vi "OCR_Setting_UI.vi"(6 "Analysis_Setting":T1={"PreProcess"=enum."*Algorithm*", "Parameter"=""}, 8 "error in (no error)":errorcluster, 9 "ProjectName":string="CDF", 10 "LstBox Refnum":refnum<vi>, 11 "Vision_Image":T4(plugin-control)) -> (0 "error out":errorcluster, 1 "Cancel?":bool, 3 "output cluster":T1={"PreProcess"=enum."*Algorithm*", "Parameter"=""})   [LabVIEW 2019]
uses:
  Controls/_UI Command Cluster/OCR_UI Command.ctl
  Controls/_UI Command Cluster/OCR_UI Command Array.ctl
  Controls/Analysis_Type.ctl
  Controls/OCR/Analysis_OCR_Setting Parameter.ctl
  Controls/Analysis_Setting.ctl
  Controls/V_Analysis_Type.ctl
  Ctrl/VisionProcessName.ctl
panel:
  in  "OCR_Setting":T3
  in  "OCRRun":bool
  in  "Done":bool
  in  "Cancel":bool
  in  "OCRTab":enum32{"Standard Setting", "Result"}(tab)
  in  "OCRLangAdd":bool
  in  "OCRLangRemove":bool
  in  "OCRSelectedLanaguage":i32(listbox)
  in  "OCRLanguage":u16(ring)
  out "OCR Result":string
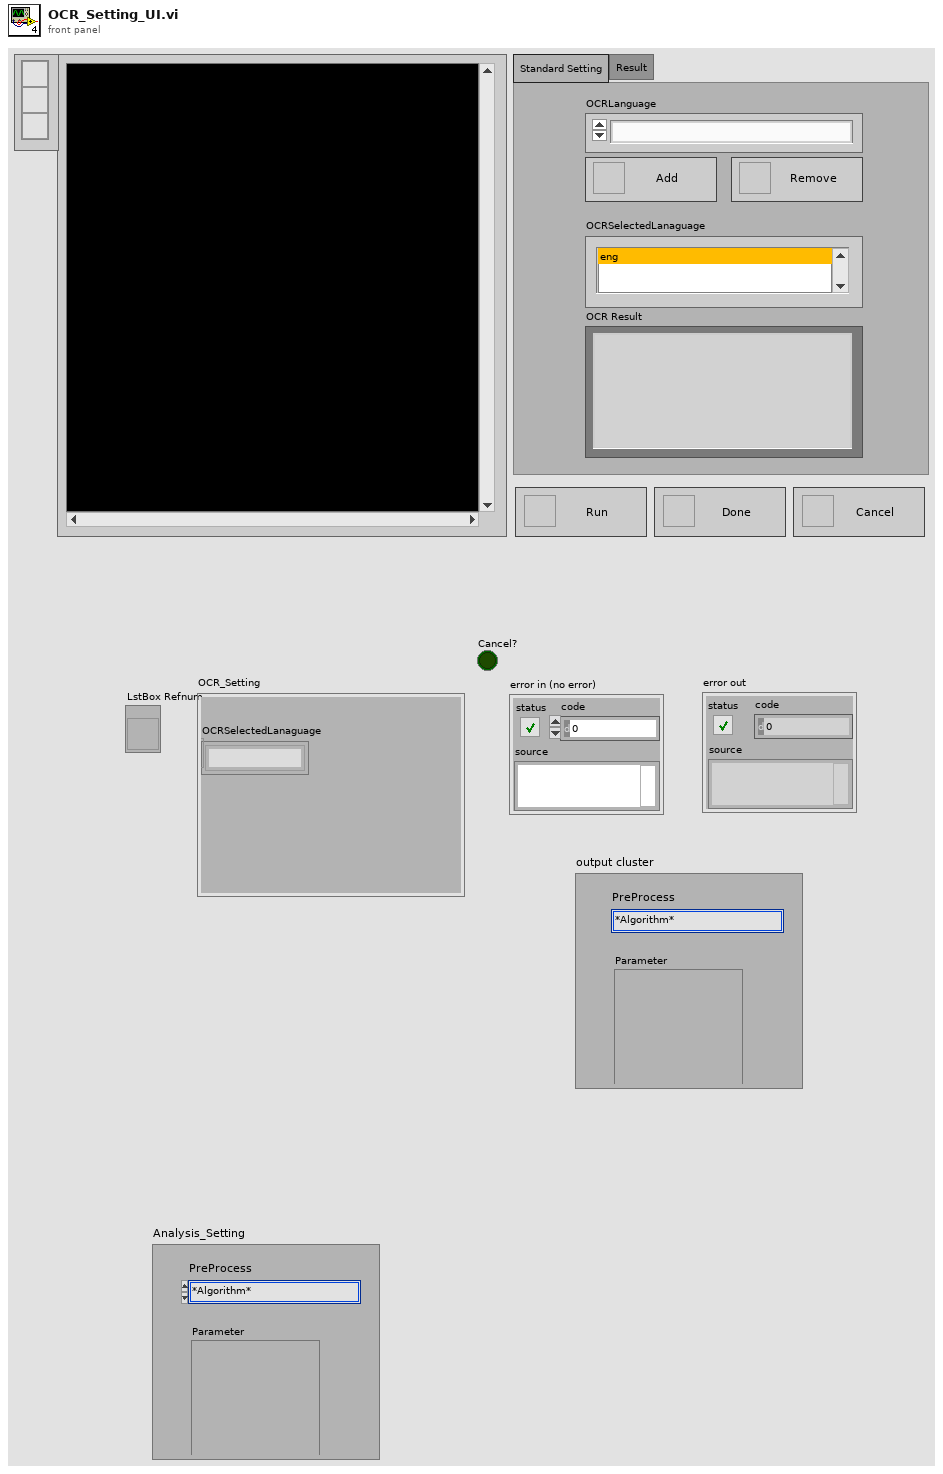
[diagram p1: front panel]
types:
  T1 = typedef "Analysis_Setting.ctl" = cluster{"PreProcess":T2, "Parameter":string}
  T2 = typedef "VisionProcessName.ctl" = enum16{"*CamParameter*", "CamAttributes", "*Preprocess*", "CG_Brightness", "C_Plane Extraction", "C_Threshold", "G_Lookup Table", "G_Threshold", "B_Image Inversion", "*Algorithm*", "CG_Histogram", "C_Color Matching", "C_Color Pattern Matching", "G_PatternMatch", "CG_Find Straight Edge", "CG_Adv. Find Straight Edge", "CG_Find Circular Edge", "G_Max Clamp", "G_Clamp (Rake)", "G_Pattern Matching"}
  T3 = typedef "Analysis_OCR_Setting Parameter.ctl" = cluster{"OCRSelectedLanaguage":string[]}
  T4 = typedef "IMAQ Image.ctl" = refnum<image>
  T5 = typedef "OCR_UI Command Array.ctl" = T6[]
  T6 = typedef "OCR_UI Command.ctl" = enum16{"Initialize", "Read Language Package", "Run", "Get Project ROI Name", "Done", "Cancel", "Add To Language", "Remove To Language", "Read Result", "Delete File", "Draw Overlay"}
  T7 = cluster{"Desired Font (Application)":enum16{"User-specified Font", "Application Font", "System Font", "Dialog Font"}, "[User-specified Font]":cluster{"Font Name":string, "Size":i16, "Strikeout?":bool, "Italic?":bool, "Underline?":bool, "Outline?":bool, "Shadow?":bool, "Bold?":bool, "Rotation Angle":dbl}, "Horizontal Alignment":i16, "Vertical Alignment":i16}
  T8 = typedef "Analysis_Type.ctl" = u16
  T9 = typedef "Analysis_Setting.ctl" = cluster{"PreProcess":T10, "Parameter":string}
  T10 = typedef "V_Analysis_Type.ctl" = enum16{"None", "C_Color Pattern Matching", "G_PatternMatching", "G_ShapeDectect", "G_GeometricMatch", "B_Area Check"}
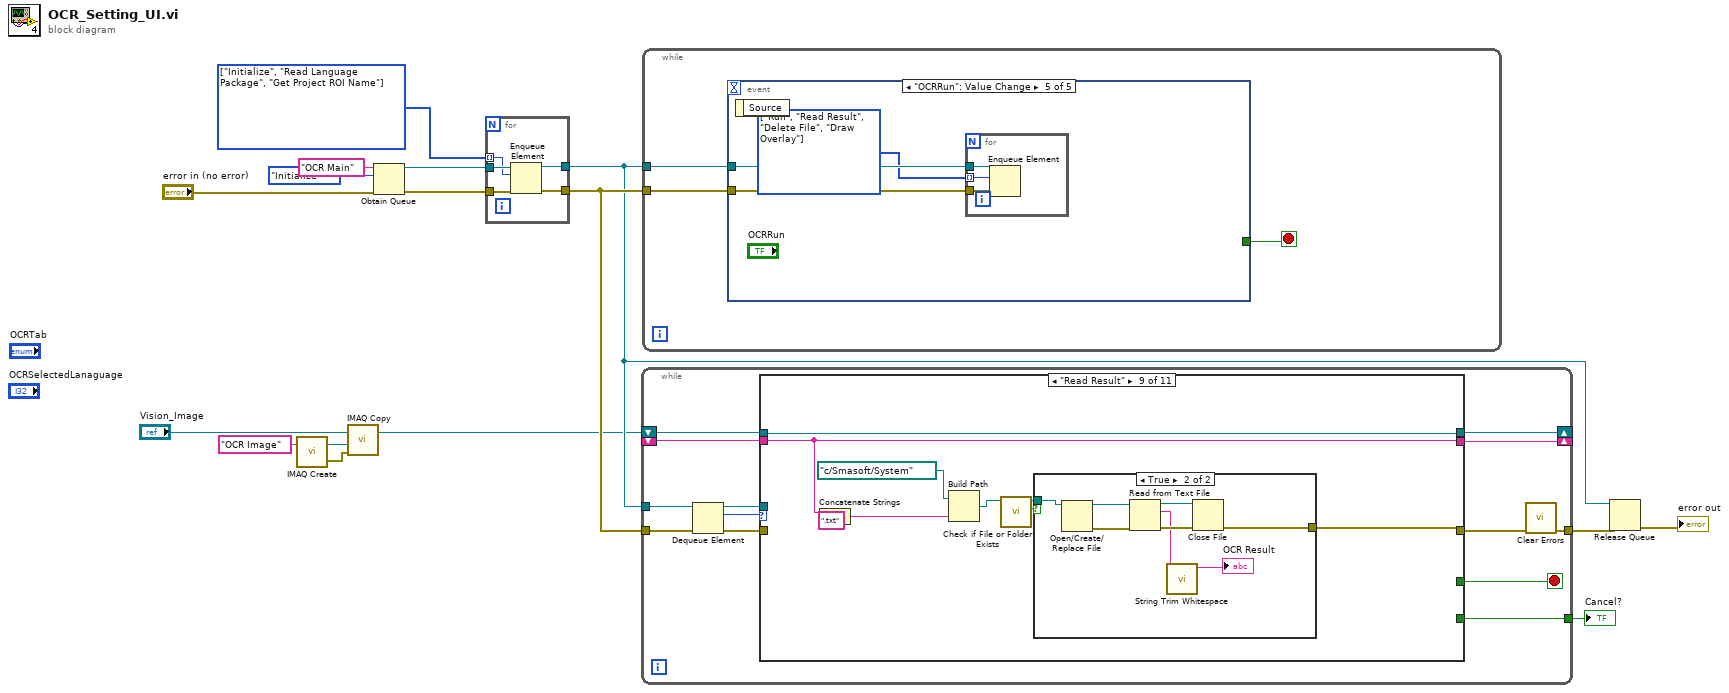
[diagram p0: block diagram]
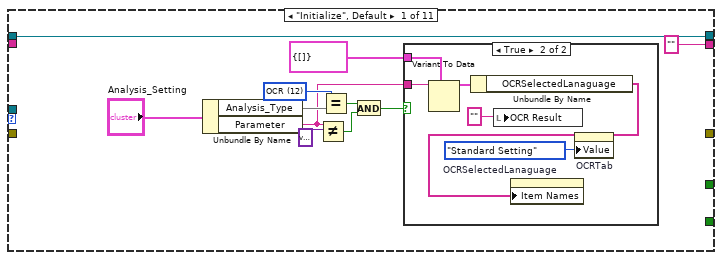
[diagram p2: hidden frame]
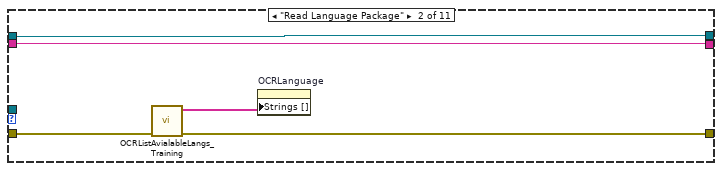
[diagram p4: hidden frame]
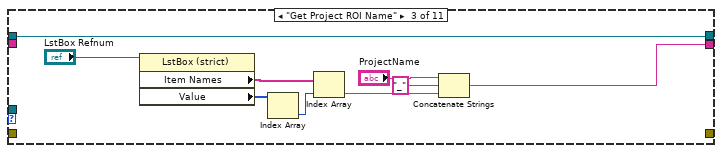
[diagram p5: hidden frame]
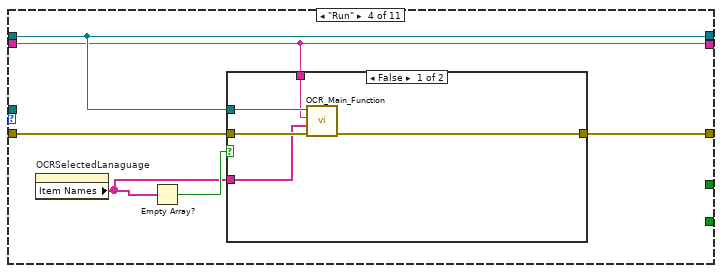
[diagram p6: hidden frame]
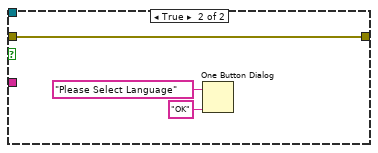
[diagram p7: hidden frame]
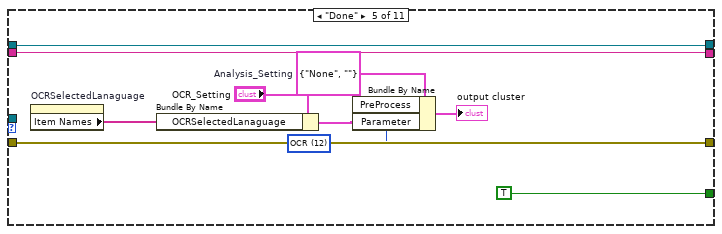
[diagram p8: hidden frame]
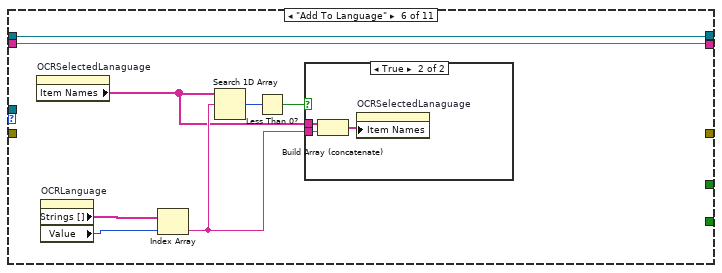
[diagram p9: hidden frame]
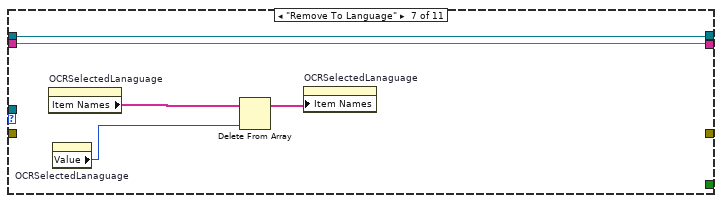
[diagram p11: hidden frame]
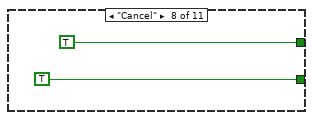
[diagram p12: hidden frame]
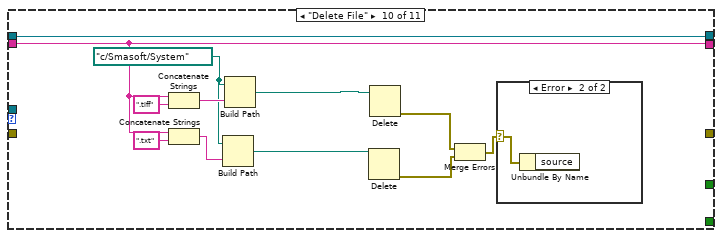
[diagram p14: hidden frame]
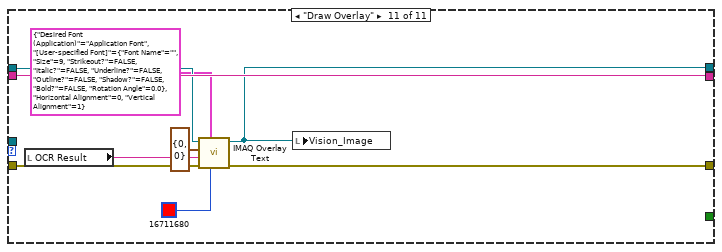
[diagram p16: hidden frame]
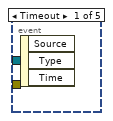
[diagram p17: hidden frame]
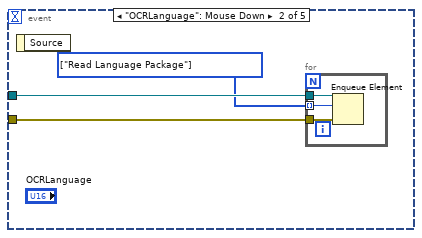
[diagram p18: hidden frame]
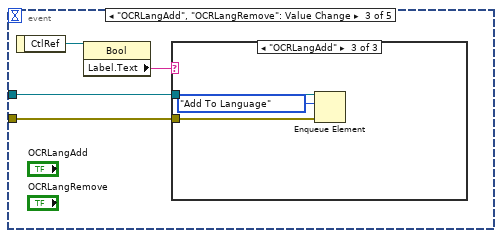
[diagram p19: hidden frame]
diagram:
  w10 = T5 [enum."Initialize", enum."Read Language Package", enum."Get Project ROI Name"] items=["Initialize", "Read Language Package", "Run", "Get Project ROI Name", "Done", "Cancel", "Add To Language", "Remove To Language", "Read Result", "Delete File", "Draw Overlay"] ("element")
  n1 = call "IMAQ Create"("Image Name"="OCR Image") -> ("New Image"=w5:T4, "error out"=w4:errorcluster)  [unwired: 4 in]
  n2 = call "IMAQ Copy"("error in (no error)"=w4, "Image Dst"=w5, "Image Src"="Vision_Image") -> ("Image Dst Out"=w2:T4)  [unwired: 3 in, 1 out]
  n3 = Obtain Queue(name (unnamed)="OCR Main", element data type=OCR_UI_Command."Initialize" ("OCR_UI Command"), error in (no error)="error in (no error)") -> (queue out=w12:refnum<queue>, error out=w11:errorcluster)  [unwired: 2 in, 1 out]
  n4 = for {
    tunnel: [w21] -> w16
    tunnel: [w20] -> w9
    tunnel: w12 -> [w19]
    tunnel: w11 -> [w18]
    tunnel: w10 -> [w17] mode=indexing
    n5 = Enqueue Element(queue=w19, element=w17, error in (no error)=w18) -> (queue out=w20:refnum<queue>, error out=w21:errorcluster)  [unwired: 1 in, 1 out]
  }
  n6 = while {
    tunnel: w16 -> [w34]
    tunnel: w9 -> [w33]
    tunnel: [w23] -> w1
    shift-right: [w27] -> _
    shift-left: _ -> [w26]
    shift-right: [w25] -> _
    shift-left: w2 -> [w28]
    tunnel: [w24] -> w7
    stop <- w29 stop-if-true
    n7 = Dequeue Element(queue=w33, error in (no error)=w34) -> (queue out=w32:refnum<queue>, element=w30:T6, error out=w31:errorcluster)  [unwired: 1 in, 1 out]
    n8 = case shown="\"Read Result\"" w30 {
      tunnel: w32 -> [_ _ _ _ _ _ _ _ _ _ _]
      tunnel: w31 -> [_ w53 _ w71 w82 _ _ _ _ _ w144]
      tunnel: [_ w52 _ w70 w82 _ _ _ w108 _ w143] -> w22
      tunnel: [_ _ _ _ TRUE _ _ TRUE _ _ _] -> w29
      tunnel: w28 -> [w45 w56 w57 w69 w89 w95 w102 _ w116 w136 w139]
      tunnel: ["" w55 w58 w68 w88 w94 w101 _ w114 w133 w146] -> w27
      tunnel: w26 -> [_ w55 _ w68 w88 w94 w101 _ w114 w133 w146]
      tunnel: [w45 w56 w57 w69 w89 w95 w102 _ w116 w136 w140] -> w25
      tunnel: [_ _ _ _ _ _ _ TRUE _ _ _] -> w24
      frame "Initialize", Default {
        w40 = T8 12 items=["None", "PatternMatch", "Edge Detection", "Barcode 1D", "Barcode 2D", "Clamp", "Clamp MAX", "Particle", "Histogram", "Straight Edge", "Circle", "Shape Detect", "OCR", "Contour", "ColorMatch"] ("x")
        n9 = Unbundle By Name("Analysis_Setting") -> ("Analysis_Type"=w41, "Parameter"=w35:string)
        n10 = Not Equal?(x=w35, y=variant) -> (x != y?=w38:bool)
        n11 = Equal?(x=w40, y=w41) -> (x = y?=w39:bool)
        n12 = And(x=w39, y=w38) -> (x .and. y?=w37:bool)
        n13 = case shown="True" w37 {
          tunnel: T3 {"OCRSelectedLanaguage"=[]} ("OCR_Setting Parameter") -> [_ w50]
          tunnel: w35 -> [_ w49]
          frame False {
          }
          frame True {
            n14 = Variant To Data(type=w50, Variant=w49) -> (data=w51:T3)  [unwired: 1 in, 1 out]
            n15 = Unbundle By Name(w51) -> ("OCRSelectedLanaguage"=w48:string[])
            n16 = local write "OCR Result"("") -> ()
            n17 = property on="OCRSelectedLanaguage" class="LstBox (strict)"("Item Names"=w48) -> ()  [unwired: 2 in, 2 out]
            n18 = property on="OCRTab" class="TabCtl (strict)"("Value"=enum32{"Standard Setting", "Result"}."Standard Setting" ("OCRTab")) -> ()  [unwired: 2 in, 2 out]
          }
        }
      }
      frame "Read Language Package" {
        n19 = call "OCRListAvialableLangs_Training.vi"("error in (no error)"=w53) -> ("error out"=w52:errorcluster, "Langs"=w54:string[])  [unwired: 9 in]
        n20 = property on="OCRLanguage" class="Ring (strict)"("Strings []"=w54) -> ()  [unwired: 2 in, 2 out]
      }
      frame "Get Project ROI Name" {
        n21 = property class="LstBox (strict)"(reference="LstBox Refnum") -> ("Item Names"=w60:string[], "Value"=w59:i32[])  [unwired: 1 in, 2 out]
        n22 = Index Array(array=w59) -> (element=w62:i32)  [unwired: 1 in]
        n23 = Index Array(array=w60, index=w62) -> (element=w63:string)
        n24 = Concatenate Strings("ProjectName", "_" ("string"), w63) -> (w58:string)
      }
      frame "Run" {
        n25 = property on="OCRSelectedLanaguage" class="LstBox (strict)"() -> ("Item Names"=w66:string[])  [unwired: 2 in, 2 out]
        n26 = Empty Array?(array=w66) -> (empty?=w67:bool)
        n27 = case shown="False" w67 {
          tunnel: w71 -> [w76 w77]
          tunnel: [w75 w77] -> w70
          tunnel: w69 -> [w74 _]
          tunnel: w68 -> [w73 _]
          tunnel: w66 -> [w72 _]
          frame False {
            n28 = call "OCR_Main_Function.vi"("error in (no error)"=w76, "Item Names"=w72, "String"=w73, "Refnum in"=w74) -> ("error out"=w75:errorcluster)  [unwired: 7 in]
          }
          frame True {
            n29 = One Button Dialog(message="Please Select Language", button name ("OK")="OK") -> ()  [unwired: 1 out]
          }
        }
      }
      frame "Done" {
        w80 = T9 {"PreProcess"=enum."None", "Parameter"=""}  # Analysis_Setting
        w81 = T8 12 items=["None", "PatternMatch", "Edge Detection", "Barcode 1D", "Barcode 2D", "Clamp", "Clamp MAX", "Particle", "Histogram", "Straight Edge", "Circle", "Shape Detect", "OCR", "Contour", "ColorMatch"] ("Analysis_Type")
        n30 = property on="OCRSelectedLanaguage" class="LstBox (strict)"() -> ("Item Names"=w85:string[])  [unwired: 2 in, 2 out]
        n31 = Bundle By Name(cluster="OCR_Setting", "OCRSelectedLanaguage"=w85) -> (w86:T3)
        n32 = Bundle By Name(cluster=w80, "PreProcess"=w81, "Parameter"=w86) -> (→"output cluster":T9)
      }
      frame "Add To Language" {
        n33 = property on="OCRSelectedLanaguage" class="LstBox (strict)"() -> ("Item Names"=w90:string[])  [unwired: 2 in, 2 out]
        n34 = property on="OCRLanguage" class="Ring (strict)"() -> ("Strings []"=w96:string[], "Value"=w97:u16)  [unwired: 2 in, 2 out]
        n35 = Index Array(array=w96, index=w97) -> (element=w93:string)
        n36 = Search 1D Array(1D array=w90, element=w93) -> (index of element=w92:i32)  [unwired: 1 in]
        n37 = Less Than 0?(x=w92) -> (x < 0?=w91:bool)
        n38 = case shown="True" w91 {
          tunnel: w93 -> [_ w99]
          tunnel: w90 -> [_ w98]
          frame False {
          }
          frame True {
            n39 = Build Array (concatenate)(w98, w99) -> (w100:string[])
            n40 = property on="OCRSelectedLanaguage" class="LstBox (strict)"("Item Names"=w100) -> ()  [unwired: 2 in, 2 out]
          }
        }
      }
      frame "Remove To Language" {
        n41 = property on="OCRSelectedLanaguage" class="LstBox (strict)"() -> ("Item Names"=w105:string[])  [unwired: 2 in, 2 out]
        n42 = property on="OCRSelectedLanaguage" class="LstBox (strict)"() -> ("Value"=w104:i32)  [unwired: 2 in, 2 out]
        n43 = Delete From Array(array=w105, index=w104) -> (array with subset deleted=w103:string[])  [unwired: 1 in, 1 out]
        n44 = property on="OCRSelectedLanaguage" class="LstBox (strict)"("Item Names"=w103) -> ()  [unwired: 2 in, 2 out]
      }
      frame "Cancel" {
      }
      frame "Read Result" {
        n45 = Concatenate Strings(w114, ".txt" ("string")) -> (w112:string)
        n46 = Build Path(base path=path "c:/Smasoft/System", name or relative path=w112) -> (appended path=w111:path)
        n47 = call <vilib>:"Check if File or Folder Exists.vi"("path"=w111) -> ("file or folder exists?"=w110:bool, "dup path"=w109:path)  [unwired: 8 in, 1 out]
        n48 = case shown="True" w110 {
          tunnel: w109 -> [_ w120]
          tunnel: [_ w119] -> w108
          frame False {
          }
          frame True {
            n49 = Open/Create/Replace File(file path (use dialog)=w120) -> (refnum out=w124:refnum<file>, error out=w123:errorcluster)  [unwired: 5 in, 1 out]
            n50 = Read from Text File(file (use dialog)=w124, error in=w123) -> (refnum out=w122:refnum<file>, text=w118:string, error out=w121:errorcluster)  [unwired: 2 in, 1 out]
            n51 = call "String Trim Whitespace.vi"("String"=w118) -> ("*(type *) &x"=→"OCR Result":string)  [unwired: 10 in]
            n52 = Close File(refnum=w122, error in=w121) -> (error out=w119:errorcluster)  [unwired: 1 out]
          }
        }
      }
      frame "Delete File" {
        w131 = path "c:/Smasoft/System"
        n53 = Concatenate Strings(w133, ".tiff" ("string")) -> (w134:string)
        n54 = Concatenate Strings(w133, ".txt" ("string")) -> (w130:string)
        n55 = Build Path(base path=w131, name or relative path=w130) -> (appended path=w125:path)
        n56 = Build Path(base path=w131, name or relative path=w134) -> (appended path=w126:path)
        n57 = Delete(path (use dialog)=w125) -> (error out=w128:errorcluster)  [unwired: 4 in, 2 out]
        n58 = Delete(path (use dialog)=w126) -> (error out=w129:errorcluster)  [unwired: 4 in, 2 out]
        n59 = Merge Errors(w129, w128) -> (w127:errorcluster)
        n60 = case shown="Error" w127 {
          selector: w127 -> [_ w137]
          frame No Error {
          }
          frame Error {
            n61 = Unbundle By Name(w137) -> ()  [unwired: 1 out]
          }
        }
      }
      frame "Draw Overlay" {
        n62 = local read "OCR Result"() -> (w145:string)
        n63 = call "IMAQ Overlay Text"("Text Color (black)"=u32 16711680, "Font, Size & Style"=T7 {"Desired Font (Application)"=enum."Application Font", "[User-specified Font]"={"Font Name"="", "Size"=9, "Strikeout?"=FALSE, "Italic?"=FALSE, "Underline?"=FALSE, "Outline?"=FALSE, "Shadow?"=FALSE, "Bold?"=FALSE, "Rotation Angle"=0.0}, "Horizontal Alignment"=0, "Vertical Alignment"=1}, "error in (no error)"=w144, "String"=w145, "Origin"=cluster{"X":i32, "Y":i32} {"X"=0, "Y"=0}, "Image"=w139) -> ("error out"=w143:errorcluster, "Image Out"=w140:T4)  [unwired: 4 in]
        n64 = local write "Vision_Image"(w140) -> ()
      }
    }
    n65 = call <vilib>:"Clear Errors.vi"("error in (no error)"=w22) -> ("error out"=w23:errorcluster)  [unwired: 5 in, 1 out]
  }
  "Cancel?" <- w7
  n66 = while {
    tunnel: w16 -> [w148]
    tunnel: w9 -> [w149]
    stop <- w147 stop-if-true
    n67 = event shown="[4] \"OCRRun\": Value Change" {
      selector: _ -> [_ _ _ _ _]
      dyn-events: _ -> [_ _ _ _ _]
      timeout: _ -> [_ _ _ _ _]
      tunnel: w149 -> [_ w152 w157 w168 w181]
      tunnel: w148 -> [_ w151 w156 w167 w180]
      tunnel: [_ _ _ w166 _] -> w147
      event Timeout {
        n68 = event-data() -> ()  [unwired: 1 in, 3 out]
      }
      event "OCRLanguage": Mouse Down {
        w150 = T5 [enum."Read Language Package"] items=["Initialize", "Read Language Package", "Run", "Get Project ROI Name", "Done", "Cancel", "Add To Language", "Remove To Language", "Read Result", "Delete File", "Draw Overlay"] ("OCR_UI Command Array")
        n69 = event-data() -> ()  [unwired: 1 in, 1 out]
        n70 = for {
          tunnel: w152 -> [w155]
          tunnel: w151 -> [w154]
          tunnel: w150 -> [w153] mode=indexing
          n71 = Enqueue Element(queue=w155, element=w153, error in (no error)=w154) -> ()  [unwired: 1 in, 3 out]
        }
      }
      event "OCRLangAdd", "OCRLangRemove": Value Change {
        n72 = event-data() -> ("CtlRef"=w159:refnum<vi>)  [unwired: 1 in]
        n73 = property class="Bool"(reference=w159) -> ("Label.Text"=w158:string)  [unwired: 1 in, 2 out]
        n74 = case shown="\"OCRLangAdd\"" w158 {
          tunnel: w157 -> [_ w162 w165]
          tunnel: w156 -> [_ w161 w164]
          frame Default {
          }
          frame "OCRLangRemove" {
            n75 = Enqueue Element(queue=w162, element=OCR_UI_Command."Remove To Language", error in (no error)=w161) -> ()  [unwired: 1 in, 3 out]
          }
          frame "OCRLangAdd" {
            n76 = Enqueue Element(queue=w165, element=OCR_UI_Command."Add To Language", error in (no error)=w164) -> ()  [unwired: 1 in, 3 out]
          }
        }
      }
      event "Done", "Cancel": Value Change {
        n77 = event-data() -> ("CtlRef"=w170:refnum<vi>)  [unwired: 1 in]
        n78 = property class="Bool"(reference=w170) -> ("Label.Text"=w169:string)  [unwired: 1 in, 2 out]
        n79 = case shown="\"Cancel\"" w169 {
          tunnel: w168 -> [_ w174 w178]
          tunnel: w167 -> [_ w173 w177]
          tunnel: [_ TRUE TRUE] -> w166
          frame Default {
          }
          frame "Cancel" {
            n80 = Enqueue Element(queue=w174, element=OCR_UI_Command."Cancel", error in (no error)=w173) -> ()  [unwired: 1 in, 3 out]
          }
          frame "Done" {
            n81 = Enqueue Element(queue=w178, element=OCR_UI_Command."Done", error in (no error)=w177) -> ()  [unwired: 1 in, 3 out]
          }
        }
      }
      event "OCRRun": Value Change {
        w179 = T5 [enum."Run", enum."Read Result", enum."Delete File", enum."Draw Overlay"] items=["Initialize", "Read Language Package", "Run", "Get Project ROI Name", "Done", "Cancel", "Add To Language", "Remove To Language", "Read Result", "Delete File", "Draw Overlay"] ("OCR_UI Command Array")
        n82 = event-data() -> ()  [unwired: 1 in, 1 out]
        n83 = for {
          tunnel: w181 -> [w184]
          tunnel: w180 -> [w183]
          tunnel: w179 -> [w182] mode=indexing
          n84 = Enqueue Element(queue=w184, element=w182, error in (no error)=w183) -> ()  [unwired: 1 in, 3 out]
        }
      }
    }
  }
  n85 = Release Queue(queue=w9, error in (no error)=w1) -> (error out=→"error out":errorcluster)  [unwired: 1 in, 2 out]
